vi "Get Output state.vi"(8 "error in":errorcluster, 11 "TEC 1090 in":refnum<class "Meerstetter TEC.lvclass">) -> (0 "error out":errorcluster, 2 "Out":u32, 3 "TEC 1090 out":refnum<class "Meerstetter TEC.lvclass">)   [LabVIEW 2014, in "Meerstetter Lib.lvlib" / "Meerstetter TEC.lvclass"]
uses:
  Meerstetter TEC.lvclass
  reusable/Session APIs/Serial/Serial Session.lvclass
  Meerstetter TEC.lvclass/Meerstetter TEC.ctl
  reusable/Session APIs/Serial/Public/Asynchronous Write.vi
  reusable/Session APIs/Serial/Public/Asynchronous Read.vi
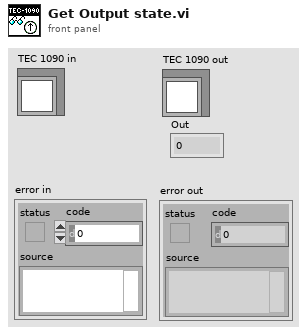
[diagram p1: front panel]
types:
  T1 = typedef "Session - Root.lvclass/Session Handle.ctl" = refnum<data-value>
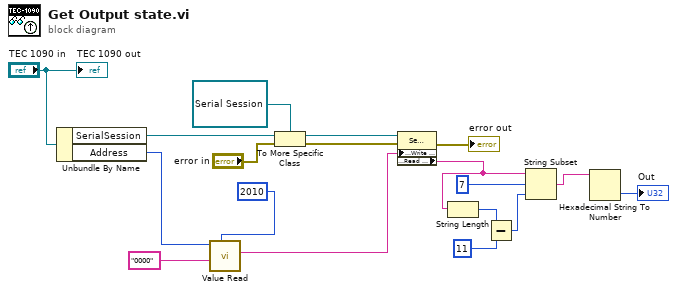
[diagram p0: block diagram]
diagram:
  n1 = Unbundle By Name("TEC 1090 in") -> ("SerialSession"=w13:T1, "Address"=w4:u8)
  n2 = call "Value Read.vi"("Read Values"=2010, "Sequence"="0000", "Address"=w4) -> ("hex integer string"=w9:string)  [unwired: 8 in]
  n3 = To More Specific Class(target class=refnum<data-value> refnum, reference=w13, error in="error in") -> (specific class reference=w11:refnum<data-value>, error out=w7:errorcluster)
  n4 = property class="Serial Session"(reference=w11, error in=w7, "Public:Write - Asynchronous"=w9) -> (error out=→"error out":errorcluster, "Public:Read - Asynchronous"=w10:string)  [unwired: 1 out]
  n5 = String Length(string=w10) -> (length=w16:i32)
  n6 = Subtract(x=w16, y=11) -> (x-y=w14:i32)
  n7 = String Subset(string=w10, offset (0)=7, length (rest)=w14) -> (substring=w2:string)
  n8 = Hexadecimal String To Number(string=w2) -> (number=→"Out":u32)  [unwired: 2 in, 1 out]
  "TEC 1090 out" <- "TEC 1090 in"
